vi "New User Event Module.vi"(8 "error in (no error)":errorcluster) -> (0 "error out":errorcluster, 3 "user event out":refnum<user-event>)   [LabVIEW 2021, in "Architecture.lvlib"]
doc: "This method creates a user event to be used to communicate between user event structures among different modules."
uses:
  Architecture.lvlib
  Typedefs/Message.ctl
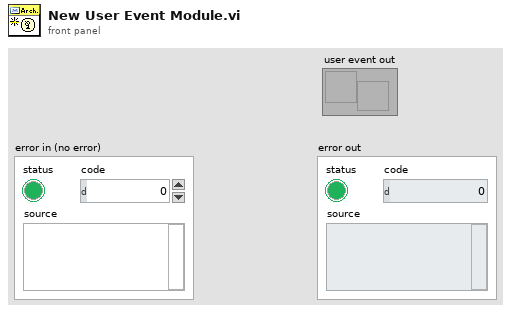
[diagram p1: front panel]
types:
  T1 = typedef "Architecture.lvlib/Message.ctl" = cluster{"Message":string, "Data":variant, "syn":bool}
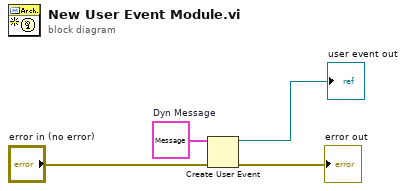
[diagram p0: block diagram]
diagram:
  w3 = T1 {"Message"="", "Data"=variant, "syn"=FALSE}  # Dyn Message
  n1 = Create User Event(user event datatype=w3, error in="error in (no error)") -> (user event=→"user event out":refnum<user-event>, error out=→"error out":errorcluster)
